vi "Untitled 1.vi"() -> ()   [LabVIEW 2023]
uses:
  Control Timer.ctl
panel:
  out "error out":errorcluster
  out "SUSENJE":bool
  out "ISPIRANJE":bool
  out "VOSKIRANJE":bool
  out "PRANJE SASIJE":bool
  out "SAMPONIRANJE":bool
  out "STATE":string
  in  "STOP":bool
  in  "Specijalno pranje":bool
  in  "Obicno pranje":bool
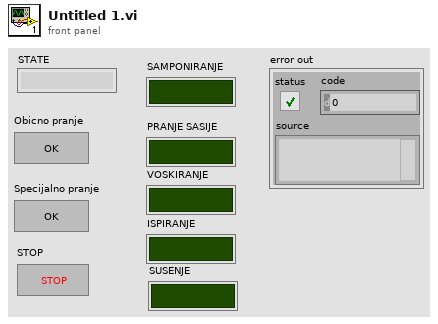
[diagram p1: front panel]
types:
  T1 = typedef "Control Timer.ctl" = enum16{"Timecheck", "Reset"}
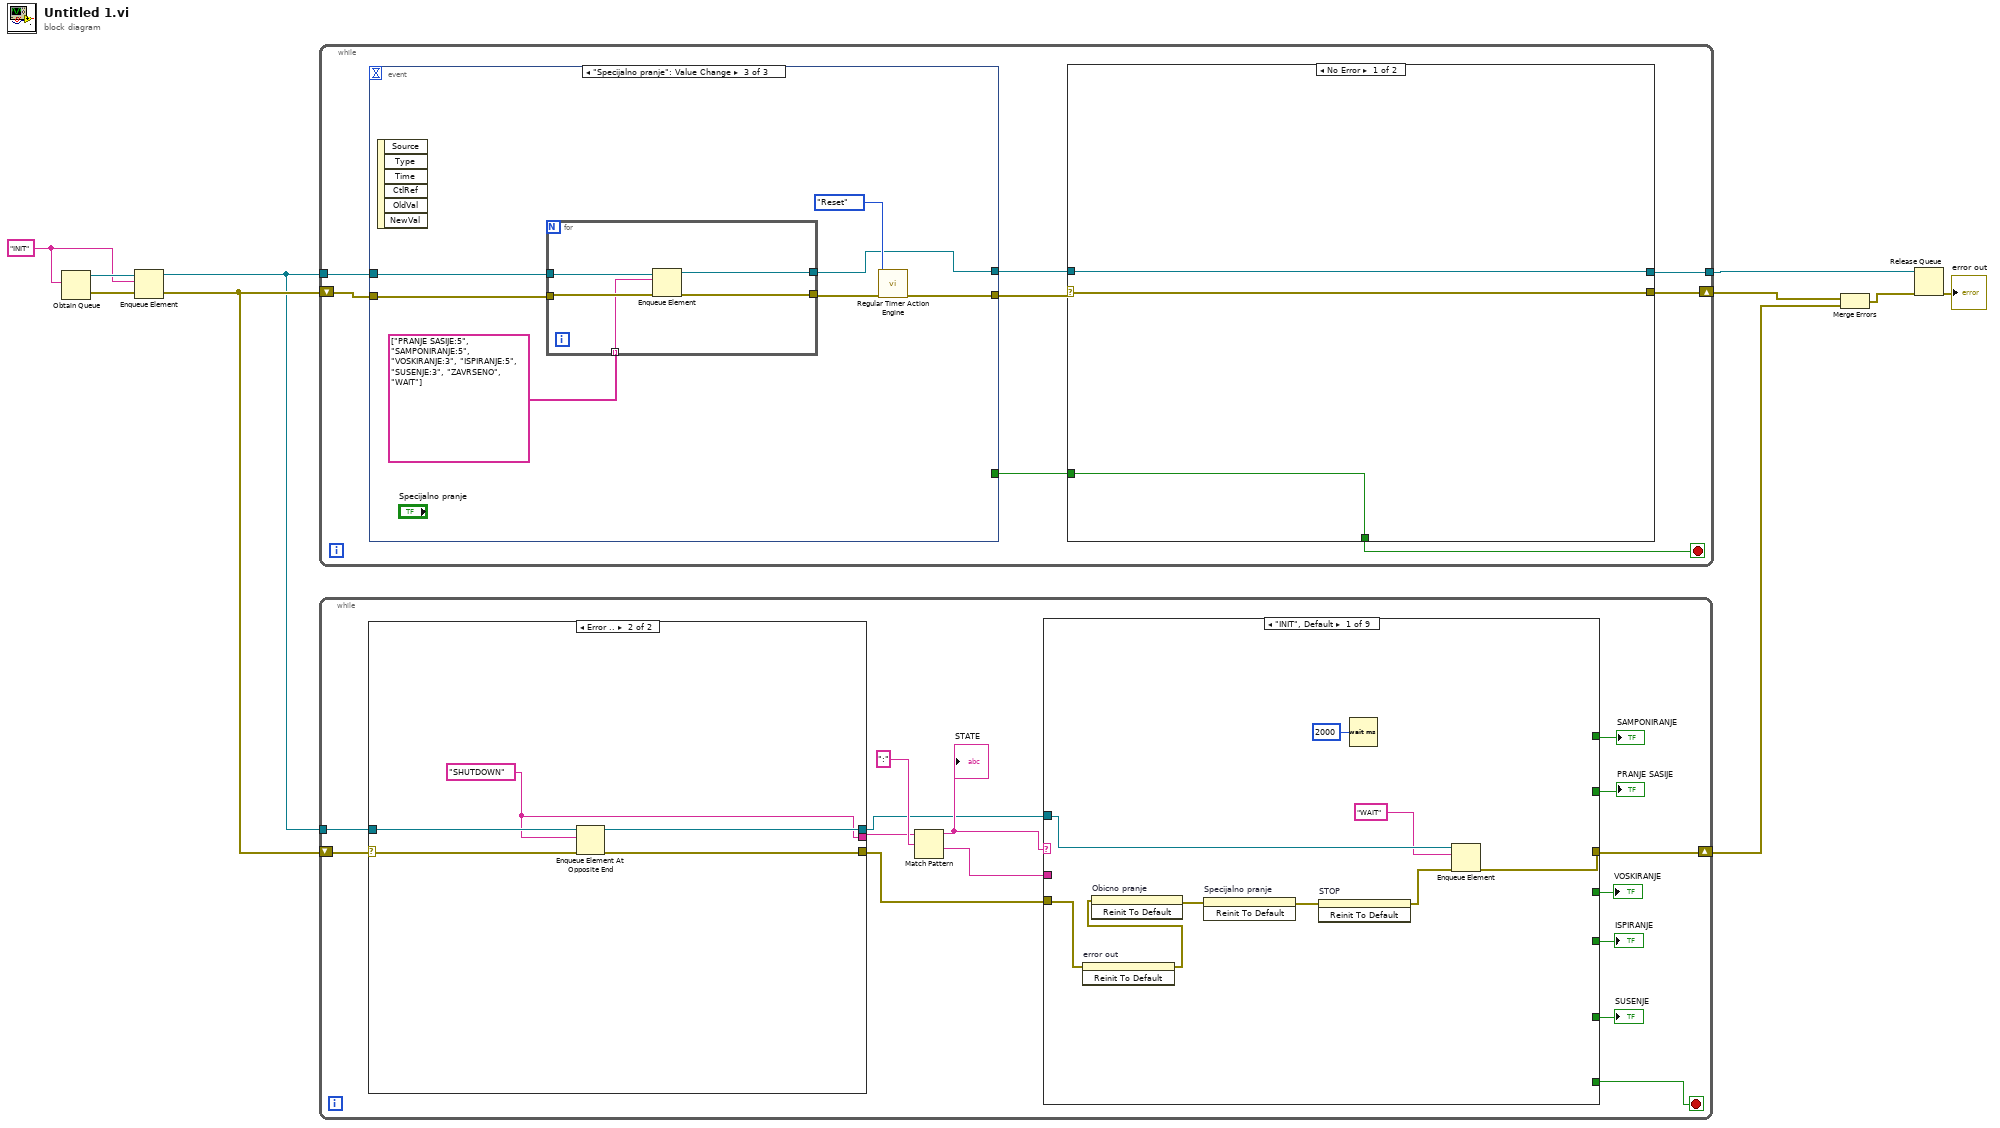
[diagram p0: block diagram]
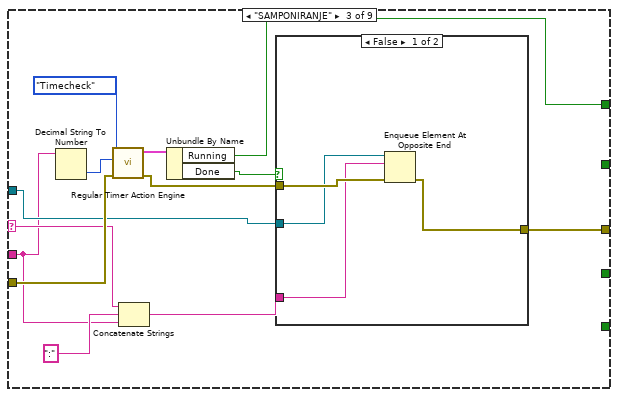
[diagram p3: hidden frame]
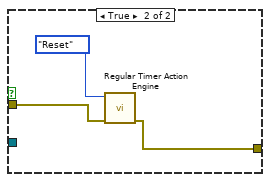
[diagram p4: hidden frame]
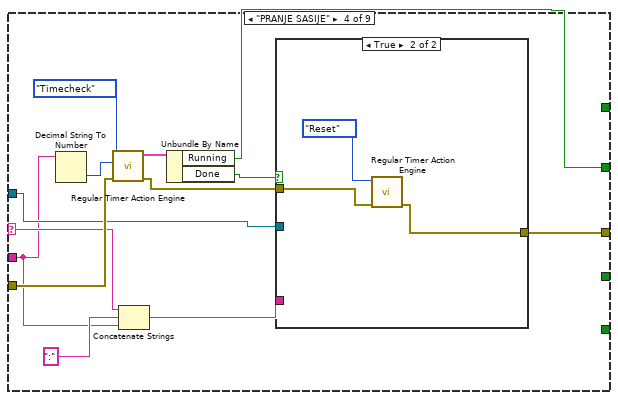
[diagram p5: hidden frame]
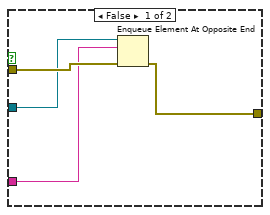
[diagram p6: hidden frame]
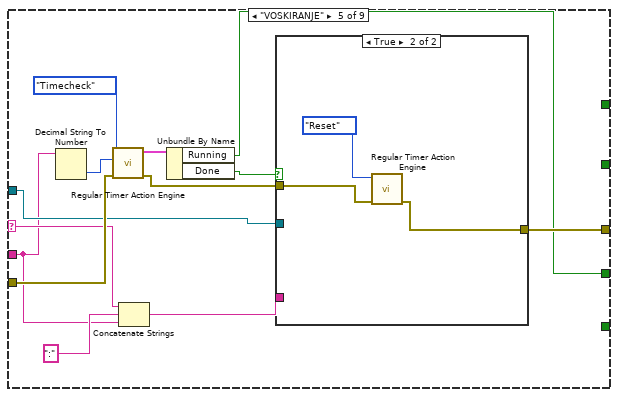
[diagram p7: hidden frame]
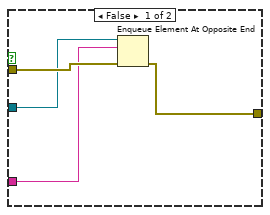
[diagram p8: hidden frame]
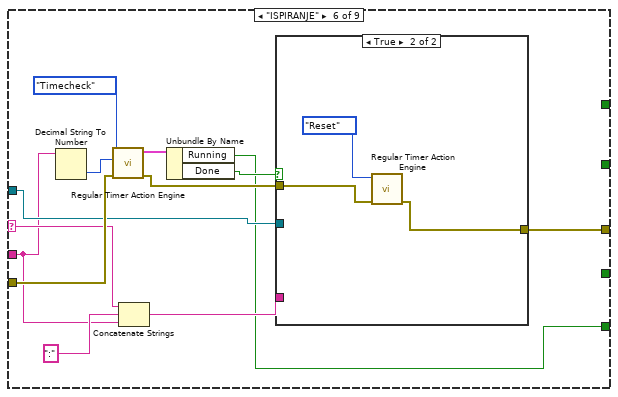
[diagram p9: hidden frame]
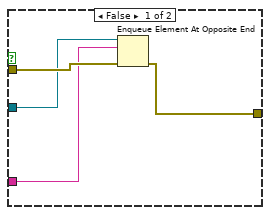
[diagram p10: hidden frame]
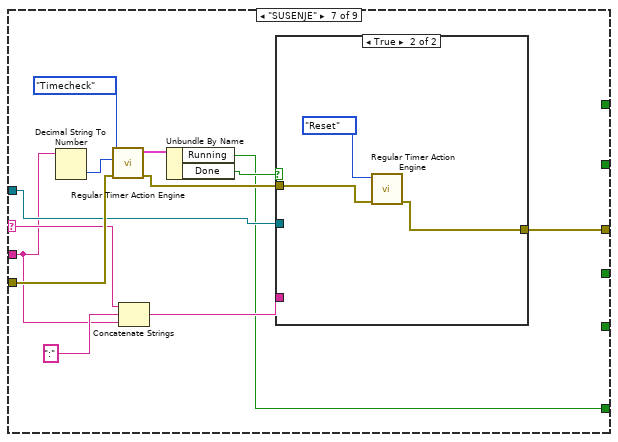
[diagram p11: hidden frame]
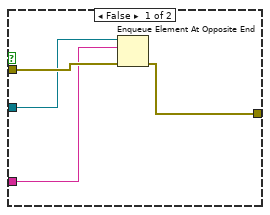
[diagram p12: hidden frame]
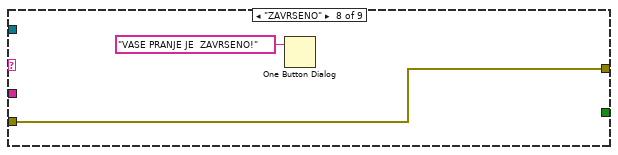
[diagram p13: hidden frame]
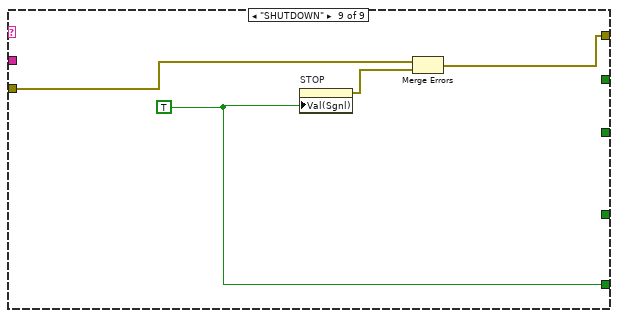
[diagram p14: hidden frame]
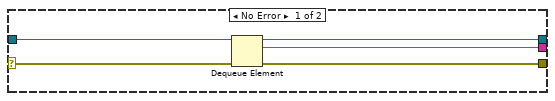
[diagram p15: hidden frame]
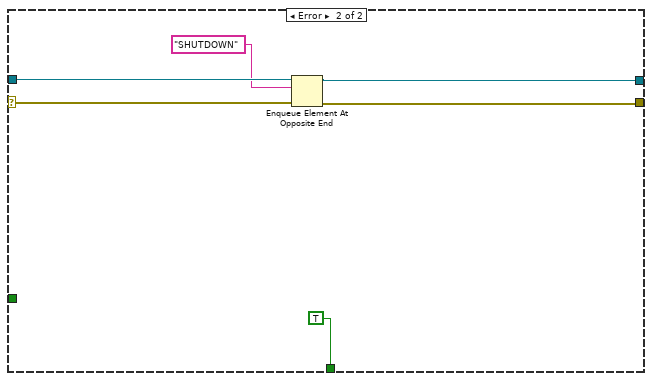
[diagram p16: hidden frame]
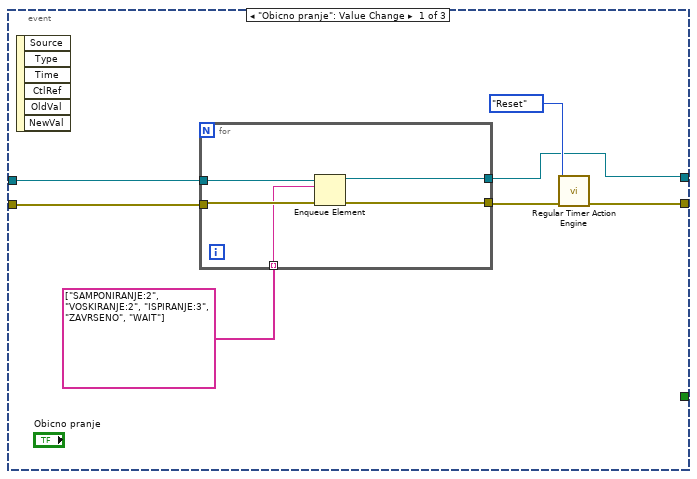
[diagram p17: hidden frame]
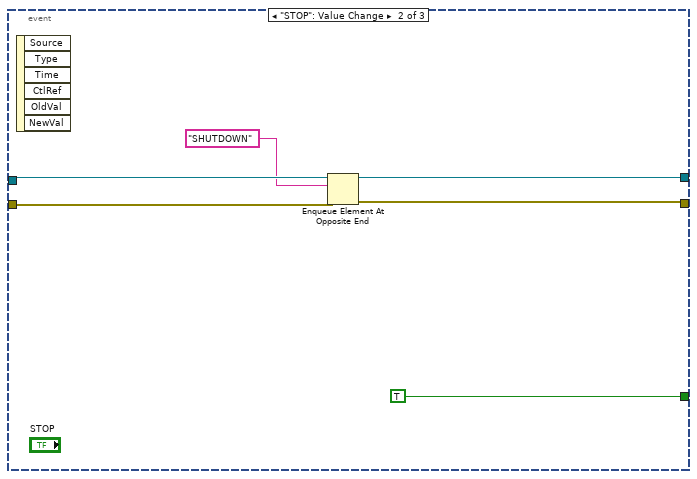
[diagram p18: hidden frame]
diagram:
  w8 = "INIT"
  n1 = Obtain Queue(element data type=w8) -> (queue out=w9:refnum<queue>, error out=w10:errorcluster)  [unwired: 4 in, 1 out]
  n2 = Enqueue Element(queue=w9, element=w8, error in (no error)=w10) -> (queue out=w6:refnum<queue>, error out=w7:errorcluster)  [unwired: 1 in, 1 out]
  n3 = while {
    tunnel: w6 -> [w24]
    shift-right: [w17] -> w3
    shift-left: w7 -> [w25]
    stop <- w11 stop-if-true
    n4 = case shown="Error .." w25 {
      selector: w25 -> [w146 w151]
      tunnel: w24 -> [w145 w150]
      tunnel: [w144 w147] -> w22
      tunnel: [w143 w148] -> w19
      tunnel: [w142 w149] -> w18
      frame No Error {
        n5 = Dequeue Element(queue=w145, error in (no error)=w146) -> (queue out=w142:refnum<queue>, element=w144:string, error out=w143:errorcluster)  [unwired: 1 in, 1 out]
      }
      frame Error {
        w147 = "SHUTDOWN"
        n6 = Enqueue Element At Opposite End(queue=w150, element=w147, error in (no error)=w151) -> (queue out=w149:refnum<queue>, error out=w148:errorcluster)  [unwired: 1 in, 1 out]
      }
    }
    n7 = Match Pattern(string=w22, regular expression=":") -> (before substring=w20:string, after substring=w21:string)  [unwired: 1 in, 2 out]
    "STATE" <- w20
    n8 = case shown="\"INIT\", Default" w20 {
      selector: w20 -> [_ _ w39 w60 w80 w100 w120 _ _]
      tunnel: w21 -> [_ _ w38 w59 w79 w99 w119 _ _]
      tunnel: w19 -> [w28 w35 w47 w67 w87 w107 w127 w136 w139]
      tunnel: w18 -> [w31 _ w41 w62 w82 w102 w122 _ _]
      tunnel: [w29 w35 w36 w57 w77 w97 w117 w136 w138] -> w17
      tunnel: [_ _ w43 _ _ _ _ _ _] -> w16
      tunnel: [_ _ _ w56 _ _ _ _ _] -> w15
      tunnel: [_ _ _ _ w76 _ _ _ _] -> w14
      tunnel: [_ _ _ _ _ w96 _ _ _] -> w13
      tunnel: [_ _ _ _ _ _ w116 _ _] -> w12
      tunnel: [_ _ _ _ _ _ _ _ w141] -> w11
      frame "INIT", Default {
        n9 = invoke on="error out" class="Clust (strict)" method="Reinit To Default"(error in=w28) -> (error out=w27:errorcluster)  [unwired: 2 in, 2 out]
        n10 = invoke on="Obicno pranje" class="Bool" method="Reinit To Default"(error in=w27) -> (error out=w34:errorcluster)  [unwired: 2 in, 2 out]
        n11 = invoke on="Specijalno pranje" class="Bool" method="Reinit To Default"(error in=w34) -> (error out=w33:errorcluster)  [unwired: 2 in, 2 out]
        n12 = invoke on="STOP" class="Bool (strict)" method="Reinit To Default"(error in=w33) -> (error out=w32:errorcluster)  [unwired: 2 in, 2 out]
        n13 = Wait (ms)(milliseconds to wait=u32 2000) -> ()  [unwired: 1 out]
        n14 = Enqueue Element(queue=w31, element="WAIT", error in (no error)=w32) -> (error out=w29:errorcluster)  [unwired: 1 in, 2 out]
      }
      frame "WAIT" {
      }
      frame "SAMPONIRANJE" {
        n15 = Decimal String To Number(string=w38) -> (number=w48:i32)  [unwired: 2 in, 1 out]
        n16 = call "Regular Timer Action Engine.vi"("Enum"=Control_Timer."Timecheck", "Time Target"=w48, "error in"=w47) -> ("Status"=w45:cluster{"Running":bool, "Done":bool}, "error out"=w42:errorcluster)  [unwired: 6 in]
        n17 = Concatenate Strings(w39, ":" ("string"), w38) -> (w37:string)
        n18 = Unbundle By Name(w45) -> ("Running"=w43:bool, "Done"=w44:bool)
        n19 = case shown="False" w44 {
          tunnel: w42 -> [w52 w55]
          tunnel: w41 -> [w51 _]
          tunnel: w37 -> [w50 _]
          tunnel: [w49 w54] -> w36
          frame False {
            n20 = Enqueue Element At Opposite End(queue=w51, element=w50, error in (no error)=w52) -> (error out=w49:errorcluster)  [unwired: 1 in, 2 out]
          }
          frame True {
            n21 = call "Regular Timer Action Engine.vi"("Enum"=Control_Timer."Reset", "error in"=w55) -> ("error out"=w54:errorcluster)  [unwired: 7 in, 1 out]
          }
        }
      }
      frame "PRANJE SASIJE" {
        n22 = Decimal String To Number(string=w59) -> (number=w68:i32)  [unwired: 2 in, 1 out]
        n23 = call "Regular Timer Action Engine.vi"("Enum"=Control_Timer."Timecheck", "Time Target"=w68, "error in"=w67) -> ("Status"=w65:cluster{"Running":bool, "Done":bool}, "error out"=w63:errorcluster)  [unwired: 6 in]
        n24 = Concatenate Strings(w60, ":" ("string"), w59) -> (w58:string)
        n25 = Unbundle By Name(w65) -> ("Running"=w56:bool, "Done"=w64:bool)
        n26 = case shown="True" w64 {
          tunnel: w63 -> [w72 w75]
          tunnel: w62 -> [w71 _]
          tunnel: w58 -> [w70 _]
          tunnel: [w69 w74] -> w57
          frame False {
            n27 = Enqueue Element At Opposite End(queue=w71, element=w70, error in (no error)=w72) -> (error out=w69:errorcluster)  [unwired: 1 in, 2 out]
          }
          frame True {
            n28 = call "Regular Timer Action Engine.vi"("Enum"=Control_Timer."Reset", "error in"=w75) -> ("error out"=w74:errorcluster)  [unwired: 7 in, 1 out]
          }
        }
      }
      frame "VOSKIRANJE" {
        n29 = Decimal String To Number(string=w79) -> (number=w88:i32)  [unwired: 2 in, 1 out]
        n30 = call "Regular Timer Action Engine.vi"("Enum"=Control_Timer."Timecheck", "Time Target"=w88, "error in"=w87) -> ("Status"=w85:cluster{"Running":bool, "Done":bool}, "error out"=w83:errorcluster)  [unwired: 6 in]
        n31 = Concatenate Strings(w80, ":" ("string"), w79) -> (w78:string)
        n32 = Unbundle By Name(w85) -> ("Running"=w76:bool, "Done"=w84:bool)
        n33 = case shown="True" w84 {
          tunnel: w83 -> [w92 w95]
          tunnel: w82 -> [w91 _]
          tunnel: w78 -> [w90 _]
          tunnel: [w89 w94] -> w77
          frame False {
            n34 = Enqueue Element At Opposite End(queue=w91, element=w90, error in (no error)=w92) -> (error out=w89:errorcluster)  [unwired: 1 in, 2 out]
          }
          frame True {
            n35 = call "Regular Timer Action Engine.vi"("Enum"=Control_Timer."Reset", "error in"=w95) -> ("error out"=w94:errorcluster)  [unwired: 7 in, 1 out]
          }
        }
      }
      frame "ISPIRANJE" {
        n36 = Decimal String To Number(string=w99) -> (number=w108:i32)  [unwired: 2 in, 1 out]
        n37 = call "Regular Timer Action Engine.vi"("Enum"=Control_Timer."Timecheck", "Time Target"=w108, "error in"=w107) -> ("Status"=w105:cluster{"Running":bool, "Done":bool}, "error out"=w103:errorcluster)  [unwired: 6 in]
        n38 = Concatenate Strings(w100, ":" ("string"), w99) -> (w98:string)
        n39 = Unbundle By Name(w105) -> ("Running"=w96:bool, "Done"=w104:bool)
        n40 = case shown="True" w104 {
          tunnel: w103 -> [w112 w115]
          tunnel: w102 -> [w111 _]
          tunnel: w98 -> [w110 _]
          tunnel: [w109 w114] -> w97
          frame False {
            n41 = Enqueue Element At Opposite End(queue=w111, element=w110, error in (no error)=w112) -> (error out=w109:errorcluster)  [unwired: 1 in, 2 out]
          }
          frame True {
            n42 = call "Regular Timer Action Engine.vi"("Enum"=Control_Timer."Reset", "error in"=w115) -> ("error out"=w114:errorcluster)  [unwired: 7 in, 1 out]
          }
        }
      }
      frame "SUSENJE" {
        n43 = Decimal String To Number(string=w119) -> (number=w128:i32)  [unwired: 2 in, 1 out]
        n44 = call "Regular Timer Action Engine.vi"("Enum"=Control_Timer."Timecheck", "Time Target"=w128, "error in"=w127) -> ("Status"=w125:cluster{"Running":bool, "Done":bool}, "error out"=w123:errorcluster)  [unwired: 6 in]
        n45 = Concatenate Strings(w120, ":" ("string"), w119) -> (w118:string)
        n46 = Unbundle By Name(w125) -> ("Running"=w116:bool, "Done"=w124:bool)
        n47 = case shown="True" w124 {
          tunnel: w123 -> [w132 w135]
          tunnel: w122 -> [w131 _]
          tunnel: w118 -> [w130 _]
          tunnel: [w129 w134] -> w117
          frame False {
            n48 = Enqueue Element At Opposite End(queue=w131, element=w130, error in (no error)=w132) -> (error out=w129:errorcluster)  [unwired: 1 in, 2 out]
          }
          frame True {
            n49 = call "Regular Timer Action Engine.vi"("Enum"=Control_Timer."Reset", "error in"=w135) -> ("error out"=w134:errorcluster)  [unwired: 7 in, 1 out]
          }
        }
      }
      frame "ZAVRSENO" {
        n50 = One Button Dialog(message="VASE PRANJE JE  ZAVRSENO!") -> ()  [unwired: 1 in, 1 out]
      }
      frame "SHUTDOWN" {
        w141 = TRUE
        n51 = property on="STOP" class="Bool (strict)"("Val(Sgnl)"=w141) -> (error out=w140:errorcluster)  [unwired: 2 in, 1 out]
        n52 = Merge Errors(w139, w140) -> (w138:errorcluster)
      }
    }
    "SAMPONIRANJE" <- w16
    "PRANJE SASIJE" <- w15
    "VOSKIRANJE" <- w14
    "ISPIRANJE" <- w13
    "SUSENJE" <- w12
  }
  n53 = while {
    shift-right: [w156] -> w4
    shift-left: w7 -> [w159]
    tunnel: w6 -> [w158]
    tunnel: [w152] -> w5
    stop <- w154 stop-if-true
    n54 = event shown="[2] \"Specijalno pranje\": Value Change" {
      selector: _ -> [_ _ _]
      dyn-events: _ -> [_ _ _]
      timeout: _ -> [_ _ _]
      tunnel: w159 -> [w175 w186 w193]
      tunnel: w158 -> [w174 w185 w192]
      tunnel: [w170 w183 w188] -> w157
      tunnel: [w169 w182 w187] -> w155
      tunnel: [_ TRUE _] -> w153
      event "Obicno pranje": Value Change {
        n55 = event-data() -> ()  [unwired: 1 in, 6 out]
        n56 = for {
          tunnel: w175 -> [w180]
          tunnel: w174 -> [w179]
          tunnel: string[] ["SAMPONIRANJE:2", "VOSKIRANJE:2", "ISPIRANJE:3", "ZAVRSENO", "WAIT"] -> [w178] mode=indexing
          tunnel: [w177] -> w172
          tunnel: [w176] -> w169
          n57 = Enqueue Element(queue=w179, element=w178, error in (no error)=w180) -> (queue out=w176:refnum<queue>, error out=w177:errorcluster)  [unwired: 1 in, 1 out]
        }
        n58 = call "Regular Timer Action Engine.vi"("Enum"=Control_Timer."Reset", "error in"=w172) -> ("error out"=w170:errorcluster)  [unwired: 7 in, 1 out]
      }
      event "STOP": Value Change {
        n59 = event-data() -> ()  [unwired: 1 in, 6 out]
        n60 = Enqueue Element At Opposite End(queue=w185, element="SHUTDOWN", error in (no error)=w186) -> (queue out=w182:refnum<queue>, error out=w183:errorcluster)  [unwired: 1 in, 1 out]
      }
      event "Specijalno pranje": Value Change {
        n61 = event-data() -> ()  [unwired: 1 in, 6 out]
        n62 = for {
          tunnel: w193 -> [w198]
          tunnel: w192 -> [w197]
          tunnel: string[] ["PRANJE SASIJE:5", "SAMPONIRANJE:5", "VOSKIRANJE:3", "ISPIRANJE:5", "SUSENJE:3", "ZAVRSENO", "WAIT"] -> [w196] mode=indexing
          tunnel: [w195] -> w190
          tunnel: [w194] -> w187
          n63 = Enqueue Element(queue=w197, element=w196, error in (no error)=w198) -> (queue out=w194:refnum<queue>, error out=w195:errorcluster)  [unwired: 1 in, 1 out]
        }
        n64 = call "Regular Timer Action Engine.vi"("Enum"=Control_Timer."Reset", "error in"=w190) -> ("error out"=w188:errorcluster)  [unwired: 7 in, 1 out]
      }
    }
    n65 = case shown="No Error" w157 {
      selector: w157 -> [w162 w167]
      tunnel: [w162 w165] -> w156
      tunnel: w155 -> [w160 w168]
      tunnel: [w161 TRUE] -> w154
      tunnel: w153 -> [w161 _]
      tunnel: [w160 w163] -> w152
      frame No Error {
      }
      frame Error {
        n66 = Enqueue Element At Opposite End(queue=w168, element="SHUTDOWN", error in (no error)=w167) -> (queue out=w163:refnum<queue>, error out=w165:errorcluster)  [unwired: 1 in, 1 out]
      }
    }
  }
  n67 = Merge Errors(w4, w3) -> (w2:errorcluster)
  n68 = Release Queue(queue=w5, error in (no error)=w2) -> (error out=→"error out":errorcluster)  [unwired: 1 in, 2 out]
